vi "Vision Processing.vi"   [LabVIEW 2011]
uses:
  GLOBALVision.vi
  GLOBALShooter.vi
  GLOBALDriver.vi
types:
  T1 = typedef "Image Type" = u32
  T2 = cluster{"axis 1 (x)":dbl, "axis 2 (y)":dbl, "axis 3 (throttle)":dbl, "axis 4":dbl, "axis 5":dbl, "axis 6":dbl}
  T3 = typedef "WPI_CameraImageSize.ctl" = enum16{"640x480", "320x240", "160x120"}
  T4 = typedef "WPI_CameraWhite Balance Values.ctl" = enum16{"Auto", "Fixed indoor", "Fixed outdoor 1", "Fixed outdoor 2", "Fixed fluorescent 1", "Fixed fluorescent 2", "Hold current"}
  T5 = typedef "WPI_CameraExposure Values.ctl" = enum16{"Auto", "Flicker-free 50 Hz", "Flicker-free 60 Hz", "Hold current"}
  T6 = cluster{"fps":i32, "compression":i32, "Image Size":T3, "Camera Resolultion":cluster{i32, i32}[], "White Balance":T4, "Exposure":T5, "Brightness":dbl, "Enable Color":bool, "Camera Address":string}
  T7 = typedef "WPI_CameraDevRef.ctl" = cluster{"Camera Address":string, "CameraStatus":errorcluster, "Acquire Image Notifier":refnum<notifier>}
  T8 = typedef "IMAQ Image.ctl" = refnum<image>
  T9 = cluster{"Position":cluster{"X":dbl, "Y":dbl}, "Distance (ft)":dbl}[]
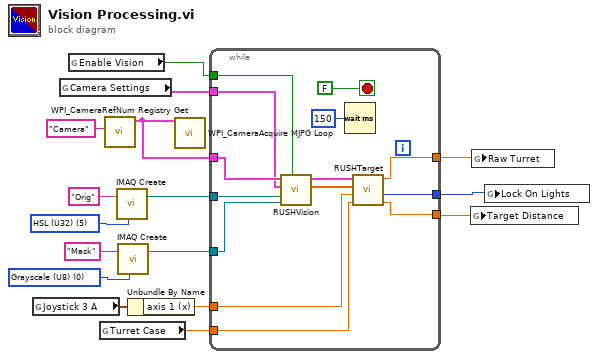
[diagram p0: block diagram]
diagram:
  w13 = T1 0 items=["Grayscale (U8)", "Grayscale (I16)", "Grayscale (SGL)", "Complex (CSG)", "RGB (U32)", "HSL (U32)", "RGB (U64)", "Grayscale (U16)"] ("Image Type")
  w15 = T1 5 items=["Grayscale (U8)", "Grayscale (I16)", "Grayscale (SGL)", "Complex (CSG)", "RGB (U32)", "HSL (U32)", "RGB (U64)", "Grayscale (U16)"] ("Image Type")
  n1 = global read "GLOBALDriver.vi" "Joystick 3 A"() -> (w4:T2)
  n2 = global read "GLOBALVision.vi" "Camera Settings"() -> (w10:T6)
  n3 = global read "GLOBALVision.vi" "Enable Vision"() -> (w9:bool)
  n4 = global read "GLOBALShooter.vi" "Turret Case"() -> (w5:dbl)
  n5 = call <vilib>:"WPI_CameraRefNum Registry Get.vi"("refnum name"="Camera") -> ("CameraDevRef"=w1:T7)  [unwired: 9 in, 1 out]
  n6 = call "IMAQ Create"("Image Name"="Orig", "Image Type"=w15) -> ("New Image"=w14:T8)  [unwired: 2 in, 2 out]
  n7 = call "IMAQ Create"("Image Name"="Mask", "Image Type"=w13) -> ("New Image"=w11:T8)  [unwired: 2 in, 2 out]
  n8 = Unbundle By Name(w4) -> ("axis 1 (x)"=w3:dbl)
  n9 = call <vilib>:"WPI_CameraAcquire MJPG Loop.vi"("CameraDevRef"=w1) -> ()  [unwired: 11 in]
  n10 = while {
    tunnel: w14 -> [w28]
    tunnel: w1 -> [w26]
    tunnel: w11 -> [w27]
    tunnel: [w23] -> w8
    tunnel: [w22] -> w7
    tunnel: [w21] -> w6
    tunnel: w10 -> [w17]
    tunnel: w9 -> [w20]
    tunnel: w5 -> [w19]
    tunnel: w3 -> [w18]
    stop <- FALSE stop-if-true
    n11 = call "RUSHVision.vi"("Enable Vision"=w20, "Mask Image"=w27, "Orig Image"=w28, "Camera Settings"=w17, "CameraDevRef"=w26) -> ("Aspect Ratio"=w24:dbl[], "Target Info"=w25:T9)  [unwired: 5 in]
    n12 = Wait (ms)(milliseconds to wait=u32 150) -> ()  [unwired: 1 out]
    n13 = call "RUSHTarget.vi"("Turret Case"=w19, "Joystick Value"=w18, "Aspect Ratio"=w24, "Target Info"=w25) -> ("Target Distance"=w21:dbl, "Lock On Lights"=w22:i32, "Raw Turret"=w23:dbl)  [unwired: 5 in]
  }
  n14 = global write "GLOBALShooter.vi" "Target Distance"(w6) -> ()
  n15 = global write "GLOBALShooter.vi" "Raw Turret"(w8) -> ()
  n16 = global write "GLOBALShooter.vi" "Lock On Lights"(w7) -> ()
